vi "Final-MurphyE-FindCOM.vi"(0 "Name of Desired\nInstrument":string="E3631A") -> (1 "Number of Active\nCOM Ports":i32, 2 "List of Active Com Ports":refnum<visa-resource-name>[](array[refnum]), 3 "Desired \nCOM Port":refnum<visa-resource-name>, 4 "Instrument\nNot Found":bool)   [LabVIEW 2018]
doc: "Searches all the active COM ports for an instrument that responds to a *idn? query with a response that includes the text given as \"Name of Desired Instrument\".\nThe list of active COM ports includes instruments that don't even respond to such queries."
uses:
  <vilib>/Instr/_visa.llb/VISA Configure Serial Port (Instr).vi
panel:
  out "Instrument Responses":string[](array[string])
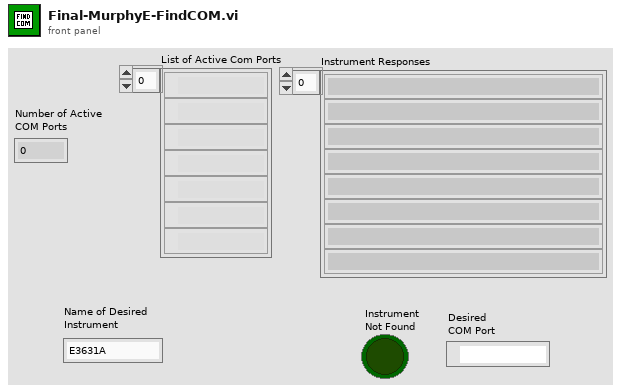
[diagram p1: front panel]
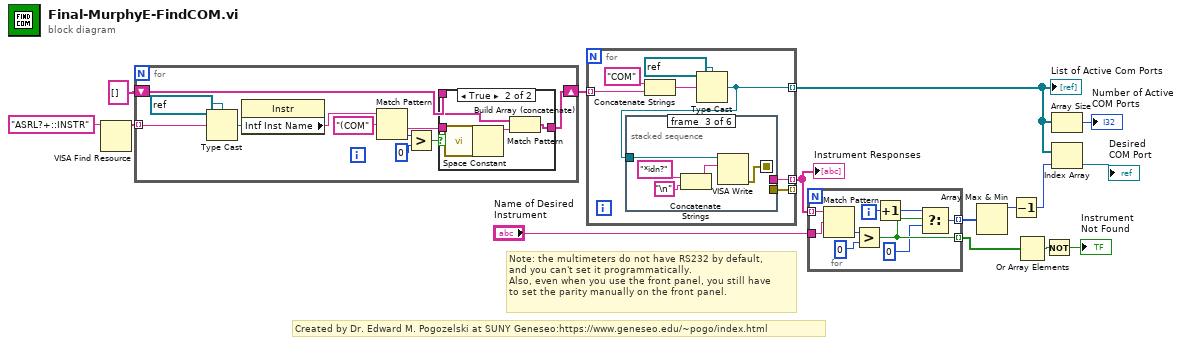
[diagram p0: block diagram]
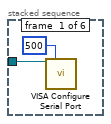
[diagram p2: hidden frame]
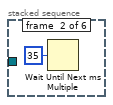
[diagram p3: hidden frame]
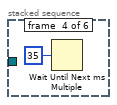
[diagram p4: hidden frame]
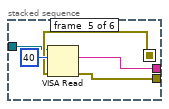
[diagram p5: hidden frame]
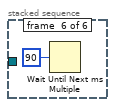
[diagram p6: hidden frame]
diagram:
  # "Created by Dr. Edward M. Pogozelski at SUNY Geneseo:https://www.geneseo.edu/~pogo/index.html"
  # "Note: the multimeters do not have RS232 by default,\nand you can't set it programmatically.\nAlso, even when you use the front panel, you still have\nto set the parity manually on the front panel."
  n1 = VISA Find Resource(11:"ASRL?+::INSTR" ("expression (\"?*\")")) -> (3:w14:string[])  [unwired: 2 in, 2 out]
  n2 = for {
    tunnel: w14 -> [w18] mode=indexing
    shift-right: [w20] -> w12
    shift-left: string[] [] -> [w21]
    n3 = Type Cast(type=refnum<visa-resource-name> "COM1" ("Com Port?"), x=w18) -> (*(type *) &x=w16:refnum<visa-resource-name>)
    n4 = property class="Instr"(reference=w16) -> ("Intf Inst Name"=w17:string)  [unwired: 1 in, 2 out]
    n5 = Match Pattern(string=w17, regular expression="(COM") -> (after substring=w22:string, offset past match=w25:i32)  [unwired: 1 in, 2 out]
    n6 = Greater?(x=w25, y=0) -> (0:w23:bool)
    n7 = case shown="True" w23 {
      tunnel: w22 -> [_ w32]
      tunnel: w21 -> [w27 w29]
      tunnel: [w27 w28] -> w20
      frame False {
      }
      frame True {
        n8 = call <vilib>:"Space Constant.vi"() -> ("String"=w31:string)
        n9 = Match Pattern(string=w32, regular expression=w31) -> (before substring=w30:string)  [unwired: 1 in, 3 out]
        n10 = Build Array (concatenate)(w29, w30) -> (w28:string[])
      }
    }
  }
  n11 = for {
    tunnel: w12 -> [w36] mode=indexing
    tunnel: [w33] -> w8 mode=indexing
    tunnel: [w35] -> w10 mode=indexing
    tunnel: [w34] -> _ mode=indexing
    n12 = Concatenate Strings("COM" ("string"), w36) -> (w37:string)
    n13 = Type Cast(type=refnum<visa-resource-name> "COM1" ("Com Port?"), x=w37) -> (*(type *) &x=w33:refnum<visa-resource-name>)
    n14 = stacked-sequence {
      seq-local: [_ _ w44 _ _ _] -> [_ _ _ _ w50 _]
      tunnel: w33 -> [w40 _ w43 _ w49 _]
      tunnel: [_ _ _ _ w52 _] -> w35
      tunnel: [_ _ _ _ w51 _] -> w34
      frame #0 {
        n15 = call-poly "VISA Configure Serial Port"("VISA resource name"=w40, "timeout (10sec)"=u32 500) -> ()  [unwired: 12 in, 2 out]
      }
      frame #1 {
        n16 = Wait Until Next ms Multiple(millisecond multiple=u32 35) -> ()  [unwired: 1 out]
      }
      frame #2 {
        n17 = Concatenate Strings("*idn?", "\n") -> (w47:string)
        n18 = VISA Write(VISA resource name=w43, write buffer=w47) -> (error out=w44:errorcluster)  [unwired: 1 in, 2 out]
      }
      frame #3 {
        n19 = Wait Until Next ms Multiple(millisecond multiple=u32 35) -> ()  [unwired: 1 out]
      }
      frame #4 {
        n20 = VISA Read(VISA resource name=w49, byte count=u32 40, error in (no error)=w50) -> (read buffer=w52:string, error out=w51:errorcluster)  [unwired: 2 out]
      }
      frame #5 {
        n21 = Wait Until Next ms Multiple(millisecond multiple=u32 90) -> ()  [unwired: 1 out]
      }
    }
  }
  "List of Active Com Ports" <- w8
  "Instrument Responses" <- w10
  n22 = for {
    tunnel: w10 -> [w62] mode=indexing
    tunnel: "Name of Desired\nInstrument" -> [w63]
    tunnel: [w58] -> w6 mode=indexing
    tunnel: [w55] -> w4 mode=indexing
    i -> [w59]
    n23 = Match Pattern(string=w62, regular expression=w63) -> (offset past match=w61:i32)  [unwired: 1 in, 3 out]
    n24 = Greater?(x=w61, y=0) -> (0:w58:bool)
    n25 = Increment(x=w59) -> (x+1=w57:i32)
    n26 = Select(t=w57, s=w58, f=0) -> (s? t:f=w55:i32)
  }
  n27 = Array Max & Min(array=w4) -> (max value=w2:i32)  [unwired: 3 out]
  n28 = Decrement(x=w2) -> (x-1=w1:i32)
  n29 = Or Array Elements(Boolean array=w6) -> (logical OR=w7:bool)
  n30 = Not(x=w7) -> (.not. x?=→"Instrument\nNot Found":bool)
  n31 = Array Size(array=w8) -> (size(s)=→"Number of Active\nCOM Ports":i32)
  n32 = Index Array(array=w8, index=w1) -> (element=→"Desired \nCOM Port":refnum<visa-resource-name>)
